vi "IMAQDevice.calculate_ImageProperties.vi"(0 "i ref in":refnum<vi>, 2 "Enum":enum16{"U8", "U16"}(ring), 5 "error in (no error)":errorcluster) -> (10 "JPEG Image":string, 11 "length per DIM service / 16 Bit":i32, 12 "Image Pixels (U8)":u8[][](array[numeric]), 13 "Image Pixels (U16)":u16[][](array[numeric]), 14 "i ref out":refnum<vi>, 15 "Image hight":i32, 16 "Image width":i32, 17 "number of DIM services":u8, 18 "total length \nDIM services / byte":i32, 19 "error out":errorcluster)   [LabVIEW 2014, in "IMAQDevice.lvlib"]
doc: "This VI converts the image information into a 2-D array of U8 (U16 not yet implemented) numbers and calculates some important properties.\n\nLicense Agreement for this software:\n\nCopyright (C)\nGesellschaft für Schwerionenforschung, GSI\nPlanckstr. 1\n64291 Darmstadt\nGermany\n\nContact: D.Beck@gsi.de \n\nThis program is free software; you can redistribute it and/or modify it under the terms of the \nGNU General Public License as published by the Free Software Foundation; either version 2 of \nthe license, or (at your option) any later version.\n\nThis program is distributed in the hope that it will be useful, but WITHOUT ANY WARRANTY; \nwithout even the implied warranty of MERCHANTABILITY or FITNESS FOR A PARTICULAR PURPOSE. See the GNU General License for more details (http://www.gnu.org).\n\nGesellschaft für Schwerionenforschung, GSI\nPlanckstr. 1, 64291 Darmstadt, Germany\nFor all questions and ideas contact: M.Richter@gsi.de, H.Brand@gsi.de or D.Beck@gsi.de.\nLast update: 16-JUN-2004"
uses:
  IMAQDevice.lvlib
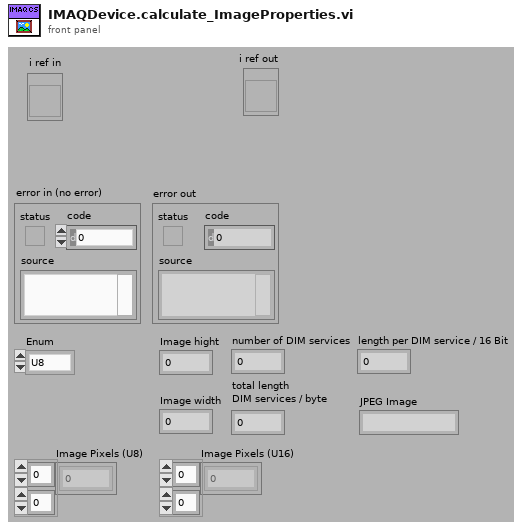
[diagram p1: front panel]
types:
  T1 = typedef "IMAQDevice.lvlib/IMAQDevice.i attribute.ctl" = cluster{"HGF_IMAQ.lvlib:HGF_IMAQDevice.lvclass":refnum<class "HGF_IMAQDevice.lvclass">, "Image":T2, "TimeStampID":i32, "Image IDs":i32[], "NumberOfImagesID":i32, "JPEG?":bool, "JPEGID":i32, "JPEG_ImageID":i32, "TriggerModeID":i32, "OffsetFromLeft":i32, "OffsetFromTop":i32, "HorizontalPixelPerMm":dbl, "VerticalPixelPerMm":dbl, "Grid":cluster{"1":cluster{i32, i32}, "2":cluster{i32, i32}, "3":cluster{i32, i32}, "4":cluster{i32, i32}}, "GridR":cluster{"1":cluster{dbl, dbl}, "2":cluster{dbl, dbl}, "3":cluster{dbl, dbl}, "4":cluster{dbl, dbl}}, "CameraTypeID":i32, "CameraInfos":cluster{"Camera Name-Array":string[], "own Camera Type":string}, "TakeMeasurement?":bool, "TriggerArmedID":i32, "Mirroring":i16, "Rotation":dbl}
  T2 = typedef "IMAQ Image.ctl" = refnum<image>
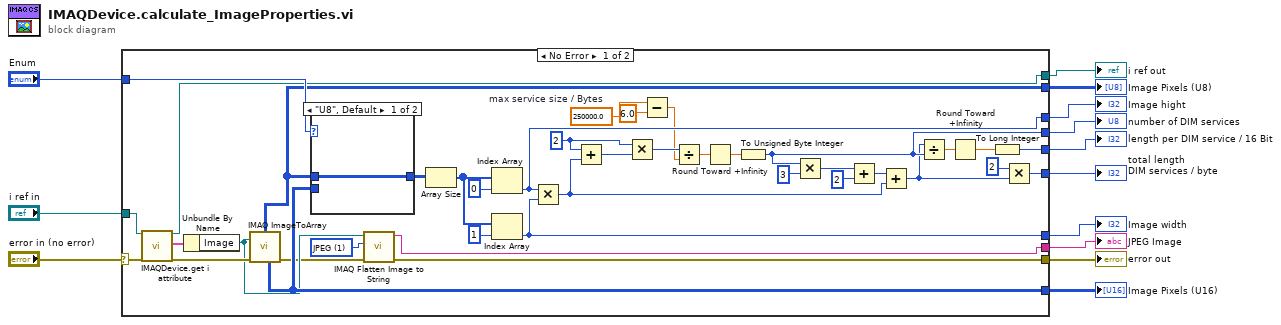
[diagram p0: block diagram]
diagram:
  n1 = case shown="No Error" "error in (no error)" {
    selector: "error in (no error)" -> [w51 w56]
    tunnel: "i ref in" -> [w52 w55]
    tunnel: [w15 w56] -> w11
    tunnel: [w40 w55] -> w10
    tunnel: [w44 _] -> w9
    tunnel: [w45 _] -> w8
    tunnel: [w38 _] -> w7
    tunnel: [w43 _] -> w6
    tunnel: [w36 _] -> w5
    tunnel: [w37 _] -> w4
    tunnel: "Enum" -> [w41 _]
    tunnel: [w39 _] -> w2
    tunnel: [w14 _] -> w1
    frame No Error {
      w18 = 1 items=["None", "JPEG", "PACKED BINARY"] ("Compression (None)")
      w21 = 250000.0  # max service size / Bytes
      w33 = 2 ("x")
      n2 = call "IMAQDevice.get i attribute.vi"("i ref in"=w52, "error in (no error)"=w51) -> ("i ref out"=w40:refnum<vi>, "i attribute"=w50:T1, "error out"=w49:errorcluster)  [unwired: 15 in]
      n3 = Unbundle By Name(w50) -> ("Image"=w17:T2)
      n4 = call "IMAQ ImageToArray"("error in (no error)"=w49, "Image"=w17) -> ("Image Pixels (U16)"=w37:u16[][], "error out"=w16:errorcluster, "Image Pixels (U8)"=w36:u8[][])  [unwired: 2 in, 2 out]
      n5 = case shown="\"U8\", Default" w41 {
        tunnel: w36 -> [w53 _]
        tunnel: [w53 w54] -> w42
        tunnel: w37 -> [_ w54]
        frame "U8", Default {
        }
        frame "U16" {
        }
      }
      n6 = call "IMAQ Flatten Image to String"("error in (no error)"=w16, "Compression (None)"=w18, "Image"=w17) -> ("error out"=w15:errorcluster, "Data String"=w14:string)  [unwired: 7 in]
      n7 = Array Size(array=w42) -> (size(s)=w46:i32[])
      n8 = Index Array(array=w46, index=0) -> (element=w45:i32)
      n9 = Index Array(array=w46, index=1) -> (element=w44:i32)
      n10 = Multiply(x=w45, y=w44) -> (x*y=w30:i32)
      n11 = Add(x=w33, y=w30) -> (x+y=w35:i32)
      n12 = Multiply(x=w33, y=w35) -> (x*y=w25:i32)
      n13 = Subtract(x=w21, y=6.0) -> (x-y=w19:dbl)
      n14 = Divide(x=w25, y=w19) -> (x/y=w23:dbl)
      n15 = Round Toward +Infinity(x=w23) -> (ceil(x): smallest int >= x=w34:dbl)
      n16 = To Unsigned Byte Integer(number=w34) -> (unsigned 8bit integer=w38:u8)
      n17 = Multiply(x=w38, y=u8 3) -> (x*y=w29:i32)
      n18 = Add(x=w29, y=u8 2) -> (x+y=w28:i32)
      n19 = Add(x=w28, y=w30) -> (x+y=w24:i32)
      n20 = Divide(x=w24, y=w38) -> (x/y=w26:dbl)
      n21 = Round Toward +Infinity(x=w26) -> (ceil(x): smallest int >= x=w22:dbl)
      n22 = To Long Integer(number=w22) -> (32bit integer=w39:i32)
      n23 = Multiply(x=2, y=w24) -> (x*y=w43:i32)
    }
    frame Error {
    }
  }
  "i ref out" <- w10
  "error out" <- w11
  "Image width" <- w9
  "Image hight" <- w8
  "number of DIM services" <- w7
  "total length \nDIM services / byte" <- w6
  "Image Pixels (U8)" <- w5
  "Image Pixels (U16)" <- w4
  "length per DIM service / 16 Bit" <- w2
  "JPEG Image" <- w1
